vi "STM Get Meta Data (TCP).vi"(8 "error in":errorcluster, 11 "Connection Info":T1) -> (0 "error out":errorcluster, 2 "Meta data":T2[](array[typedef]), 3 "Connection Info Out":T1)   [LabVIEW 2010]
doc: "Returns the meta data associated with the STM session."
uses:
  stm_TCP Connection Info.ctl
  stm_MetaDataElement.ctl
  NI STM.lvlib
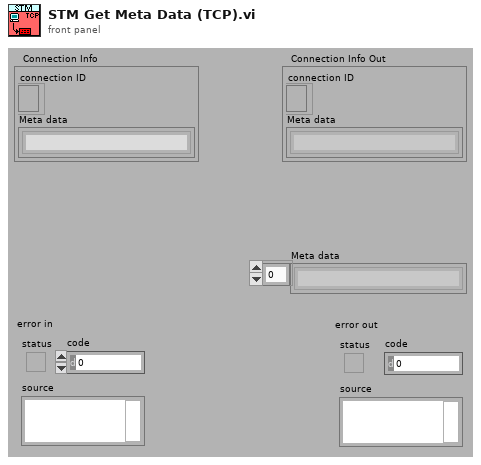
[diagram p1: front panel]
types:
  T1 = typedef "stm_TCP Connection Info.ctl" = cluster{"connection ID":refnum<k5>, "Meta data":T2[]}
  T2 = typedef "stm_MetaDataElement.ctl" = string
  T3 = typedef "NI STM.lvlib/MetaDataElement.ctl" = string
  T4 = typedef "NI STM.lvlib/TCP Connection Info.ctl" = cluster{"connection ID":refnum<k5>, "Meta data":T3[]}
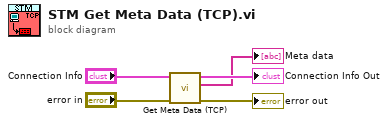
[diagram p0: block diagram]
diagram:
  n1 = call "Get Meta Data (TCP).vi"("error in"="error in", "Connection Info"="Connection Info") -> ("error out"=→"error out":errorcluster, "Meta data"=→"Meta data":T3[], "Connection Info Out"=→"Connection Info Out":T4)  [unwired: 7 in]
